vi "test_01.vi"() -> ()   [LabVIEW 2010]
panel:
  out "path":path
  out "return code":i32
  out "concatenated string":string
  out "error out":errorcluster
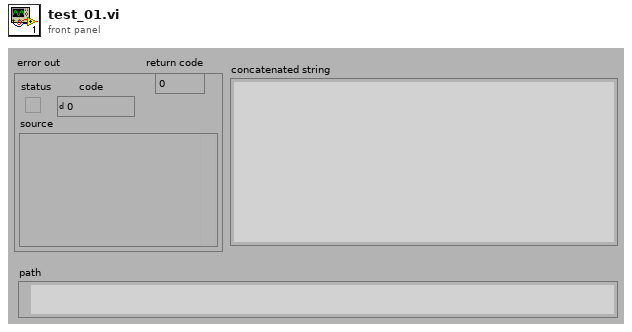
[diagram p1: front panel]
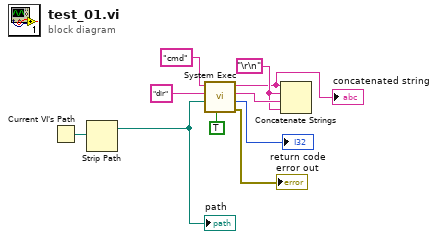
[diagram p0: block diagram]
diagram:
  w8 = "\r\n"
  n1 = Current VI's Path() -> (path=w5:path)
  n2 = Strip Path(path=w5) -> (stripped path=w1:path)  [unwired: 1 out]
  "path" <- w1
  n3 = call <vilib>:"System Exec.vi"("run minimized? (F)"=TRUE, "working directory"=w1, "standard input"="dir", "command line"="cmd") -> ("error out"=→"error out":errorcluster, "return code"=→"return code":i32, "standard error"=w9:string, "standard output"=w3:string)  [unwired: 4 in]
  "concatenated string" <- w3
  n4 = Concatenate Strings(w3, w8, w9, w8) -> ()  [unwired: 1 out]
